vi "Convert Listbox Contents to Test Parameter Cluster.vi"(10 "2D String Array":string[][](array[string])) -> (2 "Test Parameters (default)":T1)   [LabVIEW 2010, in "Core SubVIs.lvlib"]
uses:
  Core SubVIs.lvlib
  Controls/STRICT TYPE - Test Parameters.ctl
panel:
  out "Experiment Parameter Values (default)":cluster{"String":string, "value":string}[](array[cluster])
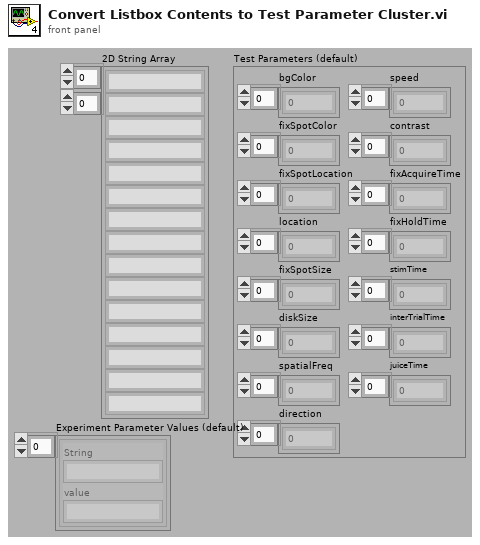
[diagram p1: front panel]
types:
  T1 = typedef "Core SubVIs.lvlib/STRICT TYPE - Test Parameters.ctl" = cluster{"bgColor":dbl[], "fixSpotColor":dbl[], "fixSpotLocation":dbl[], "location":dbl[], "fixSpotSize":dbl[], "diskSize":dbl[], "spatialFreq":dbl[], "direction":dbl[], "speed":dbl[], "contrast":dbl[], "fixAcquireTime":dbl[], "fixHoldTime":dbl[], "stimTime":dbl[], "interTrialTime":dbl[], "juiceTime":dbl[]}
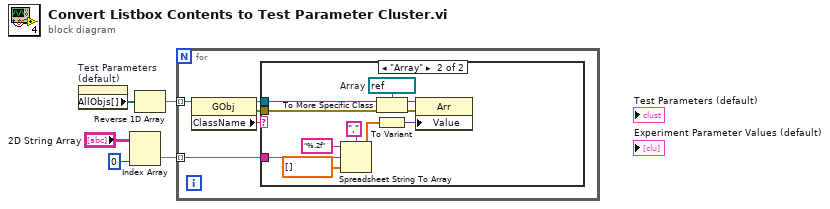
[diagram p0: block diagram]
diagram:
  n1 = property on="Test Parameters (default)" class="Clust (strict)"() -> ("AllObjs[]"=w5:refnum<vi>[])  [unwired: 2 in, 2 out]
  n2 = Index Array(array="2D String Array", index (col)=0 ("disabled index (col)")) -> (element=w1:string[])  [unwired: 1 in]
  n3 = Reverse 1D Array(array=w5) -> (reversed array=w4:refnum<vi>[])
  n4 = for {
    tunnel: w4 -> [w10] mode=indexing
    tunnel: w1 -> [w6] mode=indexing
    n5 = property class="GObj"(reference=w10) -> (reference out=w8:refnum<vi>, error out=w7:errorcluster, "ClassName"=w9:string)  [unwired: 1 in]
    n6 = case shown="\"Array\"" w9 {
      tunnel: w8 -> [_ w21]
      tunnel: w7 -> [_ w17]
      tunnel: w6 -> [_ w15]
      frame "False", Default {
      }
      frame "Array" {
        w20 = refnum<vi> refnum  # Array
        n7 = Spreadsheet String To Array(delimiter (Tab)=",", format string="%.2f", spreadsheet string=w15, array type (2D Dbl)=dbl[] []) -> (array=w11:dbl[])
        n8 = To More Specific Class(target class=w20, reference=w21, error in=w17) -> (specific class reference=w19:refnum<vi>, error out=w18:errorcluster)
        n9 = To Variant(anything=w11) -> (Variant=w16:variant)
        n10 = property class="Arr"(reference=w19, error in=w18, "Value"=w16) -> ()  [unwired: 2 out]
      }
    }
  }
